vi "GFITS_LibSetMemFits.vi"(8 "error in (no error)":errorcluster, 10 "memfits":bool) -> (0 "error out":errorcluster, 2 "return value":i32)   [LabVIEW 2016]
uses:
  c/lib/libgfits.so
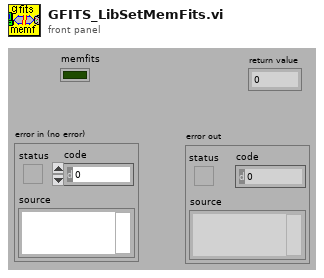
[diagram p1: front panel]
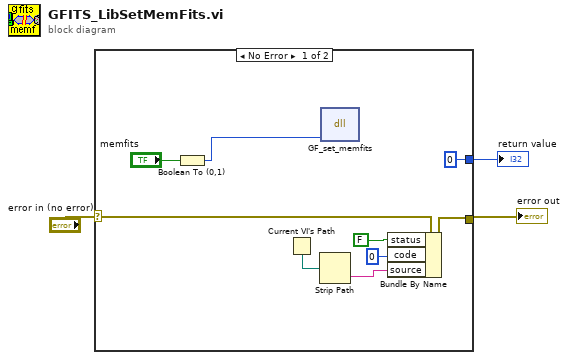
[diagram p0: block diagram]
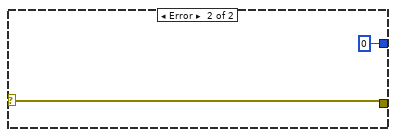
[diagram p2: hidden frame]
diagram:
  n1 = case shown="No Error" "error in (no error)" {
    selector: "error in (no error)" -> [w12 w14]
    tunnel: [0 0] -> w3
    tunnel: [w9 w14] -> w1
    frame No Error {
      n2 = Boolean To (0,1)(Boolean="memfits") -> (0, 1=w7:i16)
      n3 = Current VI's Path() -> (path=w11:path)
      n4 = Strip Path(path=w11) -> (name=w10:string)  [unwired: 1 out]
      n5 = dll-call lib="home/simager/panview/PAN/Modules/GFITS/private/c/lib/libgfits.so" fn="GF_set_memfits"("flag"=w7) -> ()  [unwired: 4 in, 3 out]
      n6 = Bundle By Name(cluster=w12, "status"=FALSE, "code"=0, "source"=w10) -> (w9:errorcluster)
    }
    frame Error {
    }
  }
  "return value" <- w3
  "error out" <- w1
